vi "spin_up_histogrammers.vi"(8 "error in (no error)":errorcluster, 9 "acq_time":i64 min=0, 10 "histo-settings":T1={"start_time(10^s)"=0.0, "stop_time(10^s)"=0.0, "start_channel"=enum."No Selection", "stop-channel"=enum."No Selection", "n_bins"=0, "Channels to\nHistogram"=[FALSE, FALSE, FALSE, FALSE, FALSE, FALSE, FALSE, FALSE]}, 11 "swabian_local_data":T3={"events"={"update_status"=refnum, "update_chart"=refnum, "update_xy"=refnum, "send_channel_data"=refnum}, "stop_q"=refnum, "tagger_reference"=refnum, "connect_button"=refnum, "counter_reference"=refnum, "tagger_stream_reference"=refnum, "log_reference"=refnum, "current_log_offset"=0, "tt20_buffer_q"=refnum, "stream_to_file_button"=refnum, "num_records"=0, "connected?"=FALSE, "plots"=refnum, "histogram_bin_edges"=[], "histogrammer"=refnum, "plot_lifetimes"=refnum, "xy_graph"=refnum, "Reference\nChannel"=enum."ch0", "trigger_channels"=[], "filter_channels"=[], "active_channels"=[], "acq_mode"=0, "Reference\nChannel"=enum."ch0", "acq_time"=0, "leftovers"={"leftover_stamps"=[], "leftover_channels"=[], "any?"=FALSE}, "sync_period_ps"=0, "raw_stream_path"=path "", "Leftovers"={"missing_sync_data"=[], "missing_events"=0}, "first_batch"=0, "first_sync_stamp"=0}) -> (0 "error out":errorcluster, 3 "swabian_local_data 2":T3={"events"={"update_status"=refnum, "update_chart"=refnum, "update_xy"=refnum, "send_channel_data"=refnum}, "stop_q"=refnum, "tagger_reference"=refnum, "connect_button"=refnum, "counter_reference"=refnum, "tagger_stream_reference"=refnum, "log_reference"=refnum, "current_log_offset"=0, "tt20_buffer_q"=refnum, "stream_to_file_button"=refnum, "num_records"=0, "connected?"=FALSE, "plots"=refnum, "histogram_bin_edges"=[], "histogrammer"=refnum, "plot_lifetimes"=refnum, "xy_graph"=refnum, "Reference\nChannel"=enum."ch0", "trigger_channels"=[], "filter_channels"=[], "active_channels"=[], "acq_mode"=0, "Reference\nChannel"=enum."ch0", "acq_time"=0, "leftovers"={"leftover_stamps"=[], "leftover_channels"=[], "any?"=FALSE}, "sync_period_ps"=0, "raw_stream_path"=path "", "Leftovers"={"missing_sync_data"=[], "missing_events"=0}, "first_batch"=0, "first_sync_stamp"=0})   [LabVIEW 2018]
uses:
  update_chart_tdef.ctl
  swabian_events_tdef.ctl
  C:/Users/SWIR TCSPC/Desktop/Swabian/lib/TTCSharp32.dll
  lib/TTCSharp32.dll
  swabian_local_data_tdef.ctl
  reference_checkbox_tdef.ctl
  swabian_buffer_tdef.ctl
  swabian_hisotgram_settings.ctl
  channel_data_tdef.ctl
  leftovers_struct.ctl
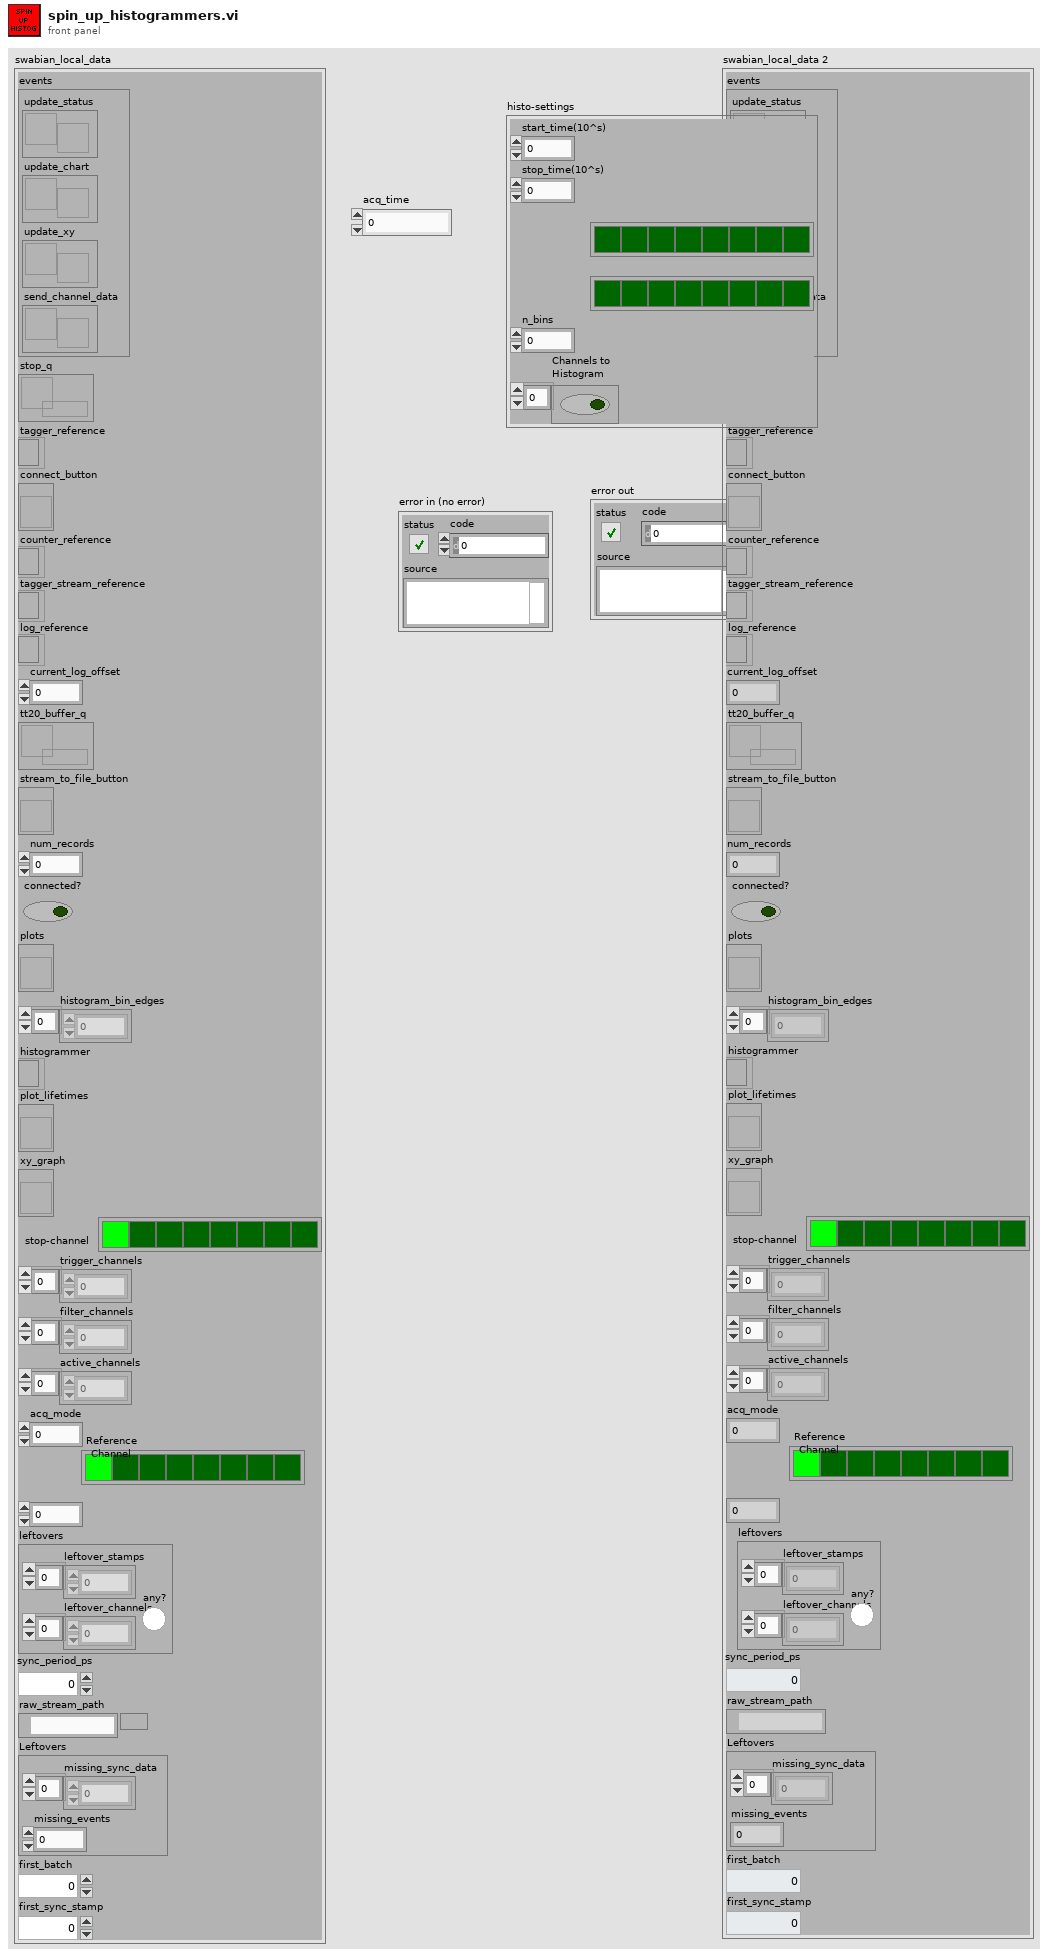
[diagram p1: front panel]
types:
  T1 = typedef "swabian_hisotgram_settings.ctl" = cluster{"start_time(10^s)":dbl, "stop_time(10^s)":dbl, "start_channel":T2, "stop-channel":T2, "n_bins":i32, "Channels to\nHistogram":bool[]}
  T2 = typedef "reference_checkbox_tdef.ctl" = enum32{"No Selection", "ch0", "ch1", "ch2", "ch3", "ch4", "ch5", "ch6", "ch7"}
  T3 = typedef "swabian_local_data_tdef.ctl" = cluster{"events":T4, "stop_q":refnum<queue>, "tagger_reference":refnum<k24>, "connect_button":refnum<vi>, "counter_reference":refnum<k24>, "tagger_stream_reference":refnum<k24>, "log_reference":refnum<file>, "current_log_offset":i64, "tt20_buffer_q":refnum<queue>, "stream_to_file_button":refnum<vi>, "num_records":u64, "connected?":bool, "plots":refnum<vi>, "histogram_bin_edges":i64[], "histogrammer":refnum<k24>, "plot_lifetimes":refnum<vi>, "xy_graph":refnum<vi>, "Reference\nChannel":T2, "trigger_channels":i32[], "filter_channels":i32[], "active_channels":i32[], "acq_mode":i32, "Reference\nChannel":T2, "acq_time":i64, "leftovers":T5, "sync_period_ps":i64, "raw_stream_path":path, "Leftovers":cluster{"missing_sync_data":u64[], "missing_events":i32}, "first_batch":i32, "first_sync_stamp":u64}
  T4 = typedef "swabian_events_tdef.ctl" = cluster{"update_status":refnum<user-event>, "update_chart":refnum<user-event>, "update_xy":refnum<user-event>, "send_channel_data":refnum<user-event>}
  T5 = typedef "leftovers_struct.ctl" = cluster{"leftover_stamps":i64[], "leftover_channels":i32[], "any?":bool}
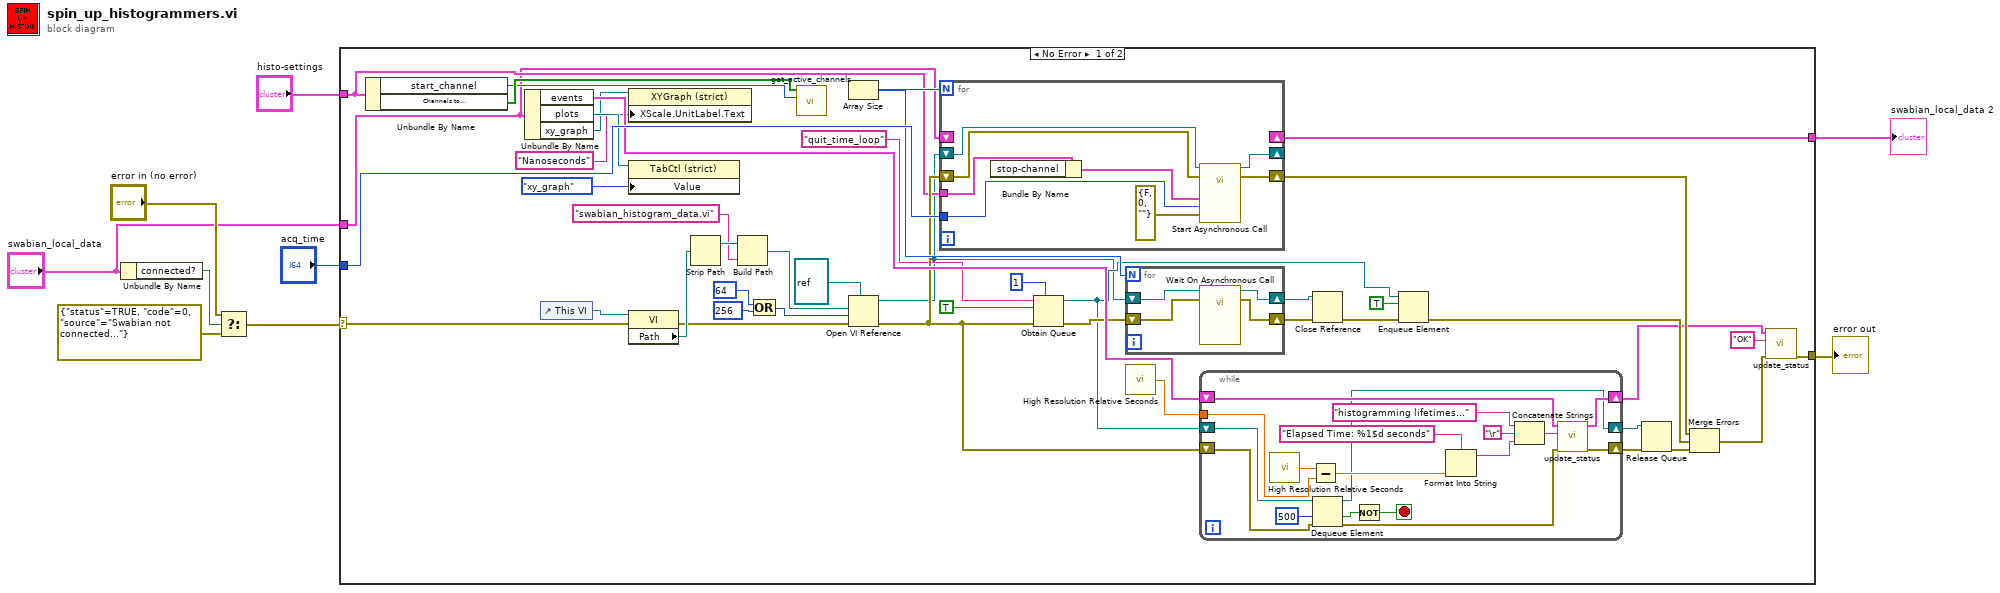
[diagram p0: block diagram]
diagram:
  n1 = Unbundle By Name("swabian_local_data") -> ("connected?"=w6:bool)
  n2 = Select(t="error in (no error)", s=w6, f=errorcluster {"status"=TRUE, "code"=0, "source"="Swabian not connected..."}) -> (s? t:f=w3:errorcluster)
  n3 = case shown="No Error" w3 {
    selector: w3 -> [w52 w84]
    tunnel: "swabian_local_data" -> [w16 w85]
    tunnel: "acq_time" -> [w44 _]
    tunnel: [w20 w84] -> w8
    tunnel: [w15 w85] -> w7
    tunnel: "histo-settings" -> [w17 _]
    frame No Error {
      n4 = Unbundle By Name(w17) -> ("start_channel"=w40:T2, "Channels to\nHistogram"=w41:bool[])
      n5 = Unbundle By Name(w16) -> ("events"=w36:T4, "plots"=w25:refnum<vi>, "xy_graph"=w11:refnum<vi>)
      n6 = control-ref of="This VI"() -> (w53:refnum<vi>)
      n7 = property class="XYGraph (strict)"(reference=w11, "XScale.UnitLabel.Text"="Nanoseconds" ("X Scale.Unit Label.Text")) -> ()  [unwired: 1 in, 2 out]
      n8 = property class="TabCtl (strict)"(reference=w25, "Value"=enum32{"chart", "xy_graph"}."xy_graph") -> ()  [unwired: 1 in, 2 out]
      n9 = property class="VI"(reference=w53, error in=w52) -> (error out=w37:errorcluster, "Path"=w51:path)  [unwired: 1 out]
      n10 = Strip Path(path=w51) -> (stripped path=w50:path)  [unwired: 1 out]
      n11 = Build Path(base path=w50, name or relative path="swabian_histogram_data.vi") -> (appended path=w48:path)
      n12 = Compound Arithmetic op=OR(64 ("options"), 256 ("options")) -> (w45:i32)
      n13 = call "get_active_channels.vi"("Reference\nChannel"=w40, "channels_to_stream"=w41) -> ()  [unwired: 8 in, 2 out]
      n14 = Array Size() -> (size(s)=w39:i32)  [unwired: 1 in]
      n15 = Open VI Reference(type specifier VI Refnum (for type only)=refnum<vi> refnum, vi path=w48, options=w45, error in (no error)=w37) -> (vi reference=w13:refnum<vi>, error out=w35:errorcluster)  [unwired: 2 in]
      n16 = for {
        N: w39 -> [_]
        shift-right: [w78] -> w43
        shift-left: w35 -> [w82]
        tunnel: w44 -> [w80]
        tunnel: w17 -> [w83]
        shift-right: [_] -> w15
        shift-left: w16 -> [_]
        shift-right: [w76] -> _
        shift-left: w13 -> [w77]
        n17 = Bundle By Name(cluster=w83) -> (w79:T1)  [unwired: 1 in]
        n18 = call-by-ref "Start Asynchronous Call"(reference=w77, error in=w82, 8:"error in (no error)"=errorcluster {"status"=FALSE, "code"=0, "source"=""} ("error in (no error)"), "acq_time"=w80, "histo-settings"=w79) -> (reference out=w76:refnum<vi>, error out=w78:errorcluster)  [unwired: 7 in, 2 out]
      }
      n19 = Obtain Queue(max queue size (-1, unlimited)=1, name (unnamed)="quit_time_loop", element data type=TRUE, error in (no error)=w35) -> (queue out=w29:refnum<queue>, error out=w34:errorcluster)  [unwired: 1 in, 1 out]
      n20 = for {
        N: w39 -> [_]
        shift-right: [w74] -> w42
        shift-left: w34 -> [w75]
        shift-right: [w72] -> w12
        shift-left: w13 -> [w73]
        n21 = call-by-ref "Wait On Asynchronous Call"(reference=w73, error in=w75) -> (reference out=w72:refnum<vi>, error out=w74:errorcluster)  [unwired: 10 in, 2 out]
      }
      n22 = call <vilib>:"High Resolution Relative Seconds.vi"() -> ("relative seconds"=w38:dbl)
      n23 = while {
        shift-right: [w67] -> w28
        shift-left: w35 -> [w60]
        tunnel: w38 -> [w70]
        shift-right: [w61] -> w19
        shift-left: w36 -> [w62]
        shift-right: [w56] -> w27
        shift-left: w29 -> [w59]
        stop <- w54 stop-if-true
        n24 = call <vilib>:"High Resolution Relative Seconds.vi"() -> ("relative seconds"=w71:dbl)
        n25 = Subtract(x=w71, y=w70) -> (x-y=w68:dbl)
        n26 = Dequeue Element(queue=w59, timeout in ms (-1)=500, error in (no error)=w60) -> (queue out=w56:refnum<queue>, timed out?=w55:bool, error out=w57:errorcluster)  [unwired: 1 out]
        n27 = Not(x=w55) -> (.not. x?=w54:bool)
        n28 = Format Into String(format string="Elapsed Time: %1$d seconds", w68) -> (resulting string=w64:string)  [unwired: 2 in, 1 out]
        n29 = Concatenate Strings("histogramming lifetimes..." ("string"), "\r", w64) -> (w63:string)
        n30 = call "update_status.vi"("error in (no error)"=w57, "status"=w63, "events"=w62) -> ("error out"=w67:errorcluster, "events_out"=w61:T4)  [unwired: 7 in]
      }
      n31 = Close Reference(reference=w12, error in (no error)=w42) -> (error out=w31:errorcluster)
      n32 = Enqueue Element(queue=w29, element=TRUE, error in (no error)=w31) -> (error out=w30:errorcluster)  [unwired: 1 in, 2 out]
      n33 = Release Queue(queue=w27, error in (no error)=w28) -> (error out=w26:errorcluster)  [unwired: 1 in, 2 out]
      n34 = Merge Errors(w43, w30, w26) -> (w21:errorcluster)
      n35 = call "update_status.vi"("error in (no error)"=w21, "status"="OK", "events"=w19) -> ("error out"=w20:errorcluster)  [unwired: 7 in, 1 out]
    }
    frame Error {
    }
  }
  "swabian_local_data 2" <- w7
  "error out" <- w8
